vi "read Hioky.vi"(8 "error in (no error)":errorcluster, 11 "VISA resource name":refnum<visa-resource-name>) -> (0 "error out":errorcluster, 1 "Measurement":dbl, 3 "VISA resource name out":refnum<visa-resource-name>)   [LabVIEW 2017]
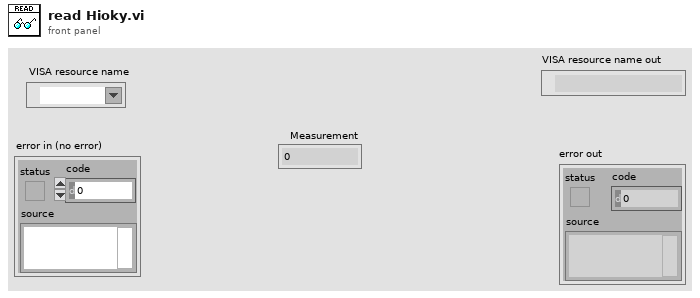
[diagram p1: front panel]
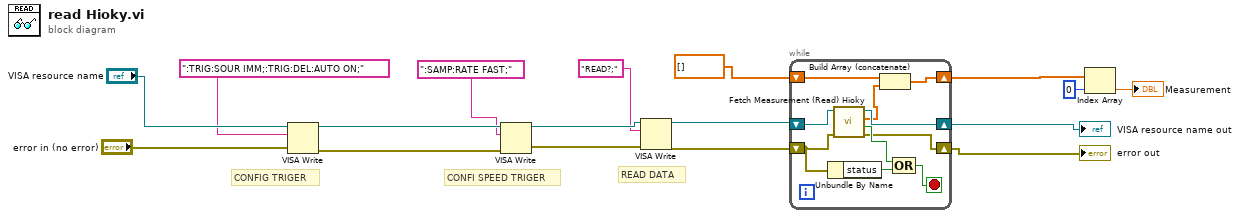
[diagram p0: block diagram]
diagram:
  # "READ DATA"
  # "CONFI SPEED TRIGER"
  # "CONFIG TRIGER"
  n1 = VISA Write(VISA resource name="VISA resource name", write buffer=":TRIG:SOUR IMM;:TRIG:DEL:AUTO ON;", error in (no error)="error in (no error)") -> (VISA resource name out=w14:refnum<visa-resource-name>, error out=w13:errorcluster)  [unwired: 1 out]
  n2 = VISA Write(VISA resource name=w14, write buffer=":SAMP:RATE FAST;", error in (no error)=w13) -> (VISA resource name out=w11:refnum<visa-resource-name>, error out=w10:errorcluster)  [unwired: 1 out]
  n3 = VISA Write(VISA resource name=w11, write buffer="READ?;", error in (no error)=w10) -> (VISA resource name out=w8:refnum<visa-resource-name>, error out=w7:errorcluster)  [unwired: 1 out]
  n4 = while {
    shift-right: [w22] -> w2
    shift-left: w8 -> [w23]
    shift-right: [w20] -> w1
    shift-left: w7 -> [w19]
    shift-right: [w25] -> w3
    shift-left: dbl[] [] -> [w24]
    stop <- w26 stop-if-true
    n5 = Unbundle By Name(w19) -> ("status"=w27:bool)
    n6 = call "Fetch Measurement (Read) Hioky.vi"("error in (no error)"=w19, "VISA resource name"=w23) -> ("error out"=w20:errorcluster, "End of Data?"=w21:bool, "Measurements"=w18:dbl[], "VISA resource name out"=w22:refnum<visa-resource-name>)  [unwired: 6 in]
    n7 = Build Array (concatenate)(w24, w18) -> (w25:dbl[])
    n8 = Compound Arithmetic op=OR(w21, w27) -> (w26:bool)
  }
  "error out" <- w1
  "VISA resource name out" <- w2
  n9 = Index Array(array=w3, index=0) -> (element=→"Measurement":dbl)
